vi "PreloadObjects2.vi"(8 "error in (no error)":errorcluster, 11 "ProgressQueue":refnum<queue>) -> (0 "error out":errorcluster)   [LabVIEW 2021, in "Application.lvclass"]
uses:
  Application.lvclass
  Interface_TAF_IApplicationConfiguration/IApplicationConfiguration/IApplicationConfiguration.lvclass
  5c5df808-c013-4a6b-85e3-bbe17662ba10.vi
  a3facc54-9779-474a-8232-32e1eb8f02f3.vi
  <vilib>/TriekselSoft/TracerLibrary/TracerLibrary/Tracer/protected/SendMessage.vi
  <vilib>/TriekselSoft/TracerLibrary/TracerLibrary/Tracer/protected/Timestamp.vi
  a3facc54-9779-474a-8232-32e1eb8f02f3.vi/f75db090-0877-4668-94fb-75c2140b1617.vi
  <vilib>/TriekselSoft/TracerLibrary/TracerLibrary/Tracer/Tracer_Level-Debug.vi
  <vilib>/TriekselSoft/TracerLibrary/TracerLibrary/Tracer/protected/Tracer_ClassAttributes.vi
  <vilib>/JDP Science/JSONtext/Variant to JSON Text.vi
  <vilib>/JDP Science/JSONtext/LVClass Serializer/JSONtext LVClass Serializer.lvclass
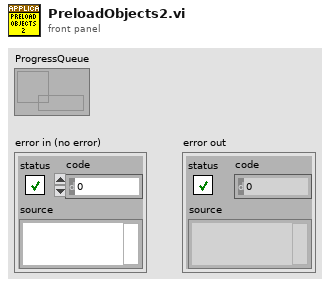
[diagram p1: front panel]
types:
  T1 = cluster{"Not found":cluster{"Name":string, "Path":string}[]}
  T2 = typedef "IApplicationConfiguration.lvclass/ObjectDataDetails.ctl" = cluster{"ObjectName":string, "ObjectType":string, "Interfaces":T3[]}
  T3 = typedef "IApplicationConfiguration.lvclass/ObjectData.ctl" = cluster{"Label":string, "ObjectName":string}
  T4 = typedef "Application.lvclass/ObjectAttributes.ctl" = cluster{"Objects":variant, "BasePath":path, "Application":refnum<class "Application.lvclass">}
  T5 = cluster{"ObjectName":string, "ObjectType":string, "error out":errorcluster}
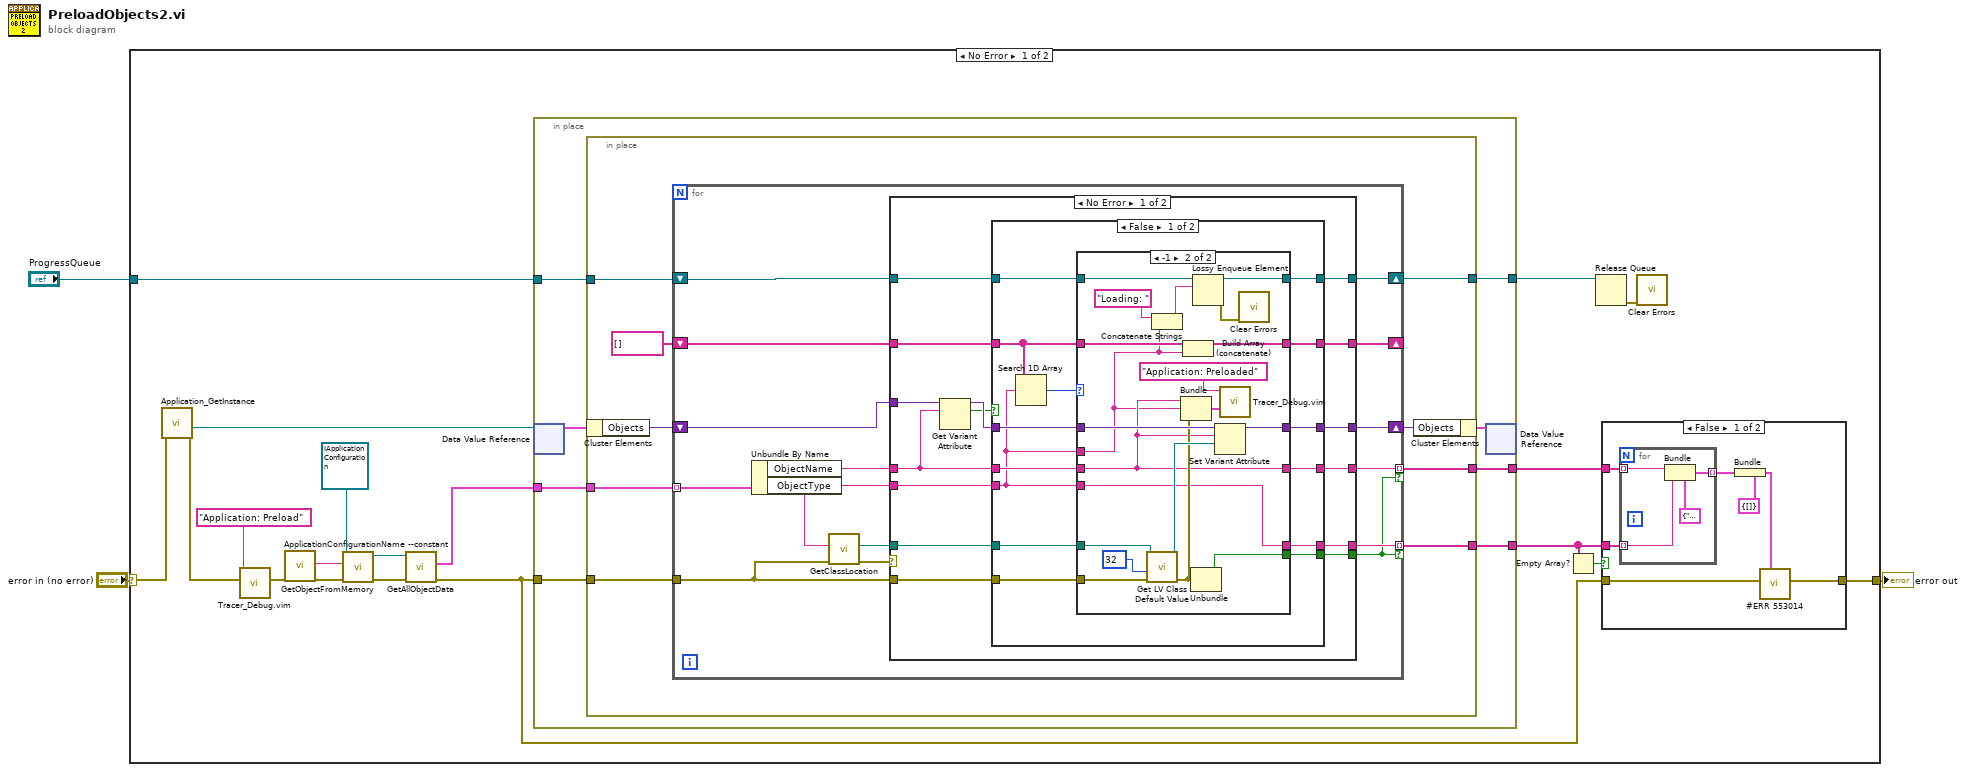
[diagram p0: block diagram]
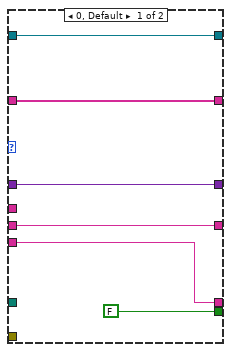
[diagram p2: hidden frame]
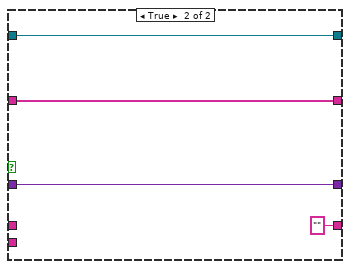
[diagram p3: hidden frame]
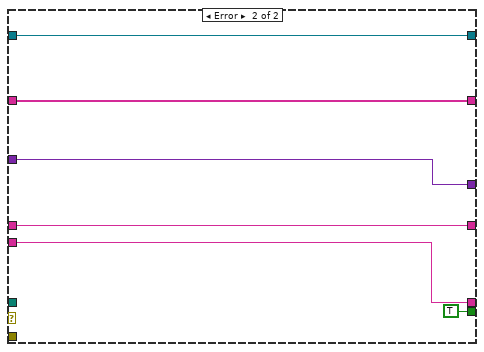
[diagram p4: hidden frame]
diagram:
  n1 = case shown="No Error" "error in (no error)" {
    selector: "error in (no error)" -> [w7 w131]
    tunnel: [w16 w131] -> w2
    tunnel: "ProgressQueue" -> [w10 _]
    frame No Error {
      n2 = call "Application_GetInstance.vi"("error in"=w7) -> ("error out"=w6:errorcluster, "DVRRefOut"=w5:refnum<data-value>)  [unwired: 6 in, 3 out]
      n3 = call "Tracer_Debug.vim"("error in (no error)"=w6, "Text"="Application: Preload") -> ("error out"=w12:errorcluster)  [unwired: 9 in]
      n4 = call "ApplicationConfigurationName --constant.vi"() -> ("AppConfigName"=w20:string)  [unwired: 10 in, 1 out]
      n5 = call "GetObjectFromMemory.vi"("error in (no error)"=w12, "ObjectName"=w20, "Type"=refnum<class "IApplicationConfiguration.lvclass"> refnum ("IApplicationStructure")) -> ("error out"=w19:errorcluster, "ObjectOut"=w18:refnum<class "IApplicationConfiguration.lvclass">)  [unwired: 7 in]
      n6 = call-dynamic "GetAllObjectData.vi"("Error In"=w19, "reference in"=w18) -> ("Error Out"=w4:errorcluster, "Objects"=w17:T2[])  [unwired: 7 in, 1 out]
      n7 = in-place {
        in-place-border: w17 -> [w29]
        in-place-border: w4 -> [w28]
        in-place-border: [w27] -> w14
        in-place-border: [w26] -> w13
        in-place-border: w10 -> [w25]
        in-place-border: [w24] -> w9
        n8 = in-place-dvr #1(w5) -> (w23:T4)  [unwired: 1 out]
        n9 = in-place {
          in-place-border: w29 -> [w38]
          in-place-border: w28 -> [w37]
          in-place-border: [w36] -> w27
          in-place-border: [w35] -> w26
          in-place-border: w25 -> [w33]
          in-place-border: [w32] -> w24
          n10 = in-place-cluster #2(w23) -> ("Objects"=w31:variant)
          n11 = for {
            tunnel: w37 -> [w43]
            tunnel: w38 -> [w45] mode=indexing
            tunnel: [w40] -> w36 mode=indexing if=w39
            tunnel: [w53] -> w35 mode=indexing if=w39
            shift-right: [w51] -> _
            shift-left: string[] [] -> [w52]
            shift-right: [w49] -> w32
            shift-left: w33 -> [w50]
            shift-right: [w47] -> w30
            shift-left: w31 -> [w48]
            n12 = Unbundle By Name(w45) -> ("ObjectName"=w46:string, "ObjectType"=w44:string)
            n13 = call "GetClassLocation.vi"("Error In"=w43, "ClassString"=w44) -> ("Error Out"=w42:errorcluster, "ClassFilePath"=w41:path)  [unwired: 8 in]
            n14 = case shown="No Error" w42 {
              tunnel: w41 -> [w68 _]
              tunnel: [w67 w115] -> w53
              tunnel: w52 -> [w66 w117]
              tunnel: [w65 w117] -> w51
              tunnel: w50 -> [w64 w118]
              tunnel: [w63 w118] -> w49
              tunnel: w48 -> [w62 w116]
              tunnel: [w61 w116] -> w47
              tunnel: w46 -> [w58 w115]
              tunnel: w43 -> [w57 _]
              tunnel: w44 -> [w56 w114]
              tunnel: [w55 w114] -> w40
              tunnel: [w54 TRUE ("status")] -> w39
              frame No Error {
                n15 = Get Variant Attribute(Variant=w62, name=w58) -> (duplicate Variant=w60:variant, found=w59:bool)  [unwired: 2 in, 2 out]
                n16 = case shown="False" w59 {
                  tunnel: w57 -> [w82 _]
                  tunnel: w68 -> [w81 _]
                  tunnel: [w80 _] -> w54
                  tunnel: w66 -> [w78 w111]
                  tunnel: [w77 w111] -> w65
                  tunnel: w58 -> [w76 _]
                  tunnel: [w75 "" ("TargetObjectName")] -> w67
                  tunnel: w64 -> [w74 w112]
                  tunnel: [w73 w112] -> w63
                  tunnel: w60 -> [w72 w110]
                  tunnel: [w71 w110] -> w61
                  tunnel: w56 -> [w69 _]
                  tunnel: [w70 _] -> w55
                  frame False {
                    n17 = Search 1D Array(1D array=w78, element=w69) -> (index of element=w79:i32)  [unwired: 1 in]
                    n18 = case shown="-1" w79 {
                      tunnel: w82 -> [_ w108]
                      tunnel: w81 -> [_ w107]
                      tunnel: [FALSE ("status") w106] -> w80
                      tunnel: w78 -> [w85 w101]
                      tunnel: w69 -> [_ w90]
                      tunnel: [w85 w100] -> w77
                      tunnel: w76 -> [w87 w91]
                      tunnel: [w87 w91] -> w75
                      tunnel: w74 -> [w86 w99]
                      tunnel: [w86 w98] -> w73
                      tunnel: w72 -> [w84 w97]
                      tunnel: [w84 w95] -> w71
                      tunnel: [w83 w89] -> w70
                      tunnel: w69 -> [w83 w89]
                      frame 0, Default {
                      }
                      frame -1 {
                        n19 = call <vilib>:"Get LV Class Default Value.vi"("error in (no error)"=w108, "options"=u32 32, "class path"=w107) -> ("error out"=w92:errorcluster, "object"=w96:refnum<class>)  [unwired: 7 in]
                        n20 = Concatenate Strings("Loading: " ("string"), w90) -> (w104:string)
                        n21 = Bundle("ObjectName"=w91, "ObjectType"=w90, "error out"=w92) -> (w93:T5)  [unwired: 1 in]
                        n22 = Build Array (concatenate)(w101, w90) -> (w100:string[])
                        n23 = Unbundle(w92) -> ("status"=w106:bool)  [unwired: 2 out]
                        n24 = Lossy Enqueue Element(queue=w99, element=w104) -> (queue out=w98:refnum<queue>, error out=w102:errorcluster)  [unwired: 1 in, 2 out]
                        n25 = Set Variant Attribute(Variant=w97, name=w91, value=w96) -> (Variant out=w95:variant)  [unwired: 1 in, 2 out]
                        n26 = call "Tracer_Debug.vim"("Data"=w93, "Text"="Application: Preloaded") -> ()  [unwired: 9 in, 1 out]
                        n27 = call <vilib>:"Clear Errors.vi"("error in (no error)"=w102) -> ()  [unwired: 5 in, 2 out]
                      }
                    }
                  }
                  frame True {
                  }
                }
              }
              frame Error {
              }
            }
          }
          n28 = in-place-cluster #2("Objects"=w30) -> (w22:T4)
        }
        n29 = in-place-dvr #1(w22) -> ()  [unwired: 2 out]
      }
      n30 = Empty Array?(array=w14) -> (empty?=w15:bool)
      n31 = Release Queue(queue=w9) -> (error out=w8:errorcluster)  [unwired: 2 in, 2 out]
      n32 = case shown="False" w15 {
        tunnel: w14 -> [w123 _]
        tunnel: w4 -> [w125 w130]
        tunnel: [w124 w130] -> w16
        tunnel: w13 -> [w122 _]
        frame False {
          n33 = for {
            tunnel: w123 -> [w127] mode=indexing
            tunnel: w122 -> [w128] mode=indexing
            tunnel: [w126] -> w121 mode=indexing
            n34 = Bundle(cluster=cluster{"Name":string, "Type":string} {"Name"="", "Type"=""}, "Name"=w128, "Type"=w127) -> (w126:cluster{"Name":string, "Type":string})
          }
          n35 = Bundle(cluster=T1 {"Not found"=[]}, "Not found"=w121) -> (w120:T1)
          n36 = call "#ERR 553014"("Data"=w120, "error in (no error)"=w125) -> ("error out"=w124:errorcluster)  [unwired: 9 in]
        }
        frame True {
        }
      }
      n37 = call <vilib>:"Clear Errors.vi"("error in (no error)"=w8) -> ()  [unwired: 5 in, 2 out]
    }
    frame Error {
    }
  }
  "error out" <- w2
